vi "AlliGator Check whether Phasor Plot needs update.vi"(9 "Error In":errorcluster) -> (1 "Error Out":errorcluster)   [LabVIEW 2021, in "AlliGator Phasor Plot.lvlib"]
doc: "Checks whether any setting that could influence the Phasor Plot has been modified."
uses:
  AlliGator Phasor Plot.lvlib
  Settings/AlliGator Settings List.ctl
  AlliGator Phasor Plot Parameters v2.ctl
  Decay Analysis/Decay Preprocessing/AlliGator Decay Preprocessing Options.ctl
  Decay Analysis/Decay Preprocessing/AlliGator Background Subtraction Parameters.ctl
  Decay Analysis/Decay Preprocessing/AlliGator Baseline Subtraction Method.ctl
  Decay Analysis/Decay Preprocessing/AlliGator Decay Preprocessing Parameters.ctl
  Graphs/XY Graph/XY Graph Plot Shift Parameters.ctl
  Graphs/XY Graph/XY Graph Plot Shift Method.ctl
  Settings/AlliGator Low Count Pixels Rejection Options.ctl
  Settings/AlliGator High Count Pixels Rejection Options.ctl
  Settings/AlliGator Gate Arithmetic.ctl
  AlliGator Phasor Plot Smoothing Options.ctl
  Arrays/Kernel Type.ctl
  Arrays/Smoothing Algorithm.ctl
  AlliGator Phasor Plot Size.ctl
  Image/Named ROI Description.ctl
  Globals, Variables, Constants/AlliGator Variables List.ctl
  Phasor Calibration/AlliGator Phasor Calibration Options.ctl
  Phasor/Phasor Calibration Type.ctl
  Phasor Calibration/AlliGator Calibration Map Algorithm.ctl
  Variant/Variant to Data/Variant to Boolean.vi
  Variant/Variant to Data/Variant to I32.vi
  Settings/AlliGator Settings.lvlib
  GUI/AlliGator GUI.lvlib
  Decay Analysis/Decay Preprocessing/AlliGator Decay Preprocessing.lvlib
  Globals, Variables, Constants/AlliGator Globals, Variables & Constants.lvlib
  Graphs/XY Graph/XY Graph Add-Ons.lvlib
  Arrays/Arrays.lvlib
  Variant/Variant to Data/Variant to Data.lvlib
  Image/Image.lvlib
  Phasor Calibration/AlliGator Phasor Calibration.lvlib
  Phasor/Phasor.lvlib
panel:
  # "see the AlliGator License on the block diagram (Ctrl+E or Window:Show Block Diagram)"
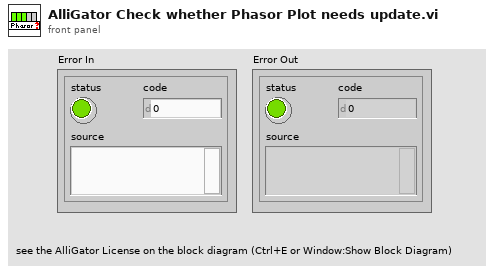
[diagram p1: front panel]
types:
  T1 = typedef "AlliGator Phasor Calibration.lvlib/AlliGator Phasor Calibration Options.ctl" = cluster{"Phasor Frequency":dbl[unit], "Phasor Calibration":cluster{"Calibration Lifetime":dbl[unit], "Calibration Type":T2, "Calibration Map Algorithm":T3, "Use Backup Calibration if needed":bool, "Backup Calibration Type":enum16{"Single Calibration", "Nearest Valid Calibration"}}}
  T2 = typedef "Phasor.lvlib/Phasor Calibration Type.ctl" = enum16{"None", "Single Phasor", "Phasor Series", "Phasor Map"}
  T3 = typedef "AlliGator Phasor Calibration.lvlib/AlliGator Calibration Map Algorithm.ctl" = enum16{"Simple Search", "Min Distance"}
  T4 = typedef "AlliGator Globals, Variables & Constants.lvlib/AlliGator Variables List.ctl" = enum16{"---- GUI ----", "GUI:Initialization Status", "GUI:State Indicators Refnum", "GUI:Original AlliGator Menu Items", "GUI:Current Action Loop State", "GUI:Script in progress", "GUI:Playback", "GUI:Loop Playback", "GUI:Search ROI Used", "GUI:Search ROI", "Decay Graph Max Legend Size", "Intensity Graph Max Legend Size", "Decay Statistics Graph Max Legend Size", "Phasor Graph Max Legend Size", "Phasor Ratio Graph Max Legend Size", "Lifetime Graph Max Legend Size", "---- Files ----", "Files:Export Dataset Frames as Individual Files", "Files:Show Batch Export Help Balloons", "Files:Frames in Dataset", "Files:ptu File Frame Start Indices", "Files:Current Frame in Dataset", "Files:Current Frame Timestamp", "Files:Dataset Loaded", "Files:Dataset Metadata", "Files:Dataset Channel", "Files:Dataset Data Description", "Files:Background Dataset Metadata", "Files:Background Dataset Channel", "Files:Background Dataset Data Description", "Files:Background File Subtraction", "Files:Background File Path", "Files:Background File Pile-up Correction", "Files:Background File Pixel Well Capacity", "Files:Background File Scaling Factor", "Files:Current Dataset Load Settings", "Files:Dataset Path", "Files:ICCD-specific Information", "Files:Macrotime Gate Separation", "------ Python Plugins ------", "Python Plugins:Information", "Python Plugins:Python Session", "Python Plugins:Valid Python Session?", "---- Source Image ----", "Source Image:ROIs", "Source Image:Current ROI", "Source Image:ROI Event Refnum", "X_Source Image Display Range", "X_Source Image Palette Information", "X_Type of Displayed Image", "X_Time Gate Slider", "Source Image:Palette List", "Source Image:Scale", "Source Image:ROI Overlay Color", "Source Image:Overlay to Erase", "Source Image:Is Displayed Image Accumulated", "Source Image:White Light Image Modified", "Source Image:Mask Image Modified", "---- Image Profile Window ----", "Image Profile:Window Event Refnum", "Image Profile:IntensityType", "Image Profile:Intensity Average Type", "Image Profile:Intensity-weighted SDV", "Image Profile:Box Profile Type", "Image Profile:Window Open", "Image Profile:Plotted Fit Parameter", "------ Phasor Graph -------", "Phasor Graph:Show Line", "---- Phasor Plot ---", "Phasor Plot:Parameters Changed", "Phasor Plot:FLI Dataset Modified since last Calculation", "Phasor Harmonics Data", "Selected Phasor Harmonics", "Phasor Harmonic Manager Event Refnum", "Phasor Plot:ROIs", "Phasor Plot:Current ROI", "Phasor Plot:ROI Event Refnum", "Phasor Plot:Image Reference Points", "Phasor Plot:Computed", "Phasor Plot:Palette Information", "Phasor Plot:Palette List", "Phasor Plot:Phasor Ratio Palette Information", "Phasor Plot:Phasor Ratio Palette List", "Phasor Plot:Image Scale", "Phasor Plot:Image Overlay to Erase", "Phasor Plot:Image Elements to Update", "Phasor Plot:Current Calculation Parameters", "Phasor Plot:Current Calibration Options", "Phasor Plot:Reset Cumulated Phasor Plot", "Phasor Plot:Reference 1", "Phasor Plot:Lifetime Reference 1", "Phasor Plot:Reference 1 Frequency", "Phasor Plot:Reference 2", "Phasor Plot:Lifetime Reference 2", "Phasor Plot:Reference 2 Frequency", "---- Decay Analysis ----", "Number of Selected Decays to Fit", "LS Fit Results", "LAR Fit Results", "BS Fit Results", "Last Decay Max - Min", "Best Fit Parameters", "Best Fit Parameter Names", "Actual Size X", "Actual Size Y", "Binning X", "Binning Y", "Actual # Gates", "Dataset Number", "Gates to...", "Gates Skipped", "Gates to keep", "Gate Step", "Gate Separation", "Reversed Gates", "Pile-up Correction", "Pixel Well Capacity", "Background Subtracted", "Background Subtraction Method", "Background Definition Range", "Background File (deprecated)", "Number of Dataset Accumulated", "Array of Accumulated Dataset Paths", "Do Averaged Datasets", "Destination File Path", "Process Plot Target", "Use 1/D as Phasor Frequency", "---- Decay Fit Parameter Map -----", "Decay Fit Parameter Map:Palette Information", "Decay Fit Parameter Map:Palette List", "---- Parameter Map ----", "Parameter Map:Palette Information", "Parameter Map:Palette List", "------- Local Decay Window ---------", "Local Decay Graph Window:Event Refnum", "Local Decay Graph Window:Use normalized IRF for convolution", "----- Miscellaneous ----", "Misc:Skippable Dialog Windows Status"}
  T5 = typedef "AlliGator Phasor Plot.lvlib/AlliGator Phasor Plot Parameters v2.ctl" = cluster{"Phasor Frequency":dbl[unit], "Decay Preprocessing Options & Parameters":T6, "FLI Dataset Modified":bool, "Source Image Settings":cluster{"Low Count Pixels Rejection Options":T12, "High Count Pixels Rejection Options":T13}, "Data Information":cluster{"Gate Width":dbl[unit], "Gate Separation":dbl[unit], "Step (Gate Separation)":i32, "Laser Period":dbl[unit], "SYNC Period":dbl[unit], "Channel Name":u16, "Channel Arithmetic":T14, "Pile-up Correction":bool, "Pixel Well Capacity":u32, "Dataset Scaling Factor":dbl}, "Phasor Plot":cluster{"Phasor Plot Smoothing Options":T15, "Phasor Plot Size":T18, "Selected Image ROI(s)":bool, "All Image ROIs":bool, "Selected Source Image ROI":i32, "Source Image ROIs":T19[]}}
  T6 = typedef "AlliGator Decay Preprocessing.lvlib/AlliGator Decay Preprocessing Options.ctl" = cluster{"Background Subtraction Parameters":T7, "Decay Preprocessing Parameters":T9, "Preprocessing Steps Order":string[]}
  T7 = typedef "AlliGator Decay Preprocessing.lvlib/AlliGator Background Subtraction Parameters.ctl" = cluster{"Background Definition Range":cluster{"Min Gate":dbl[unit], "Max Gate":dbl[unit]}, "Baseline Subtraction Method":T8, "Background Subtraction?":bool, "Background File":path, "Background Constant":dbl, "Background Scaling Factor":dbl, "Background Pile-up Correction":bool, "Background Pixel Well Capacity":u32}
  T8 = typedef "AlliGator Decay Preprocessing.lvlib/AlliGator Baseline Subtraction Method.ctl" = enum16{"Mean", "Min", "Square Gated Single-Exponential", "File", "Constant"}
  T9 = typedef "AlliGator Decay Preprocessing.lvlib/AlliGator Decay Preprocessing Parameters.ctl" = cluster{"Background Subtraction":bool, "Straighten Decay":bool, "Reverse Gates":bool, "1-Normalized Decay":bool, "Smoothen Decay":bool, "Smoothing Parameter":dbl, "Shift Decay":bool, "Decay Shift Parameters":T10, "Extrapolate Decay":bool, "Additional Points":u32, "Head Fraction":dbl, "Pixel-Normalize Decay":bool, "Use Periodicity":bool, "Use Cursors":bool, "Tail Fraction":dbl, "Use Decay Pre-Processing":bool, "Fold Decay":bool, "# Folds":u32, "[0-1]-Normalized Decay":bool}
  T10 = typedef "XY Graph Add-Ons.lvlib/XY Graph Plot Shift Parameters.ctl" = cluster{"Type":T11, "Shift":dbl[unit], "Threshold":dbl, "Rotate":bool}
  T11 = typedef "XY Graph Add-Ons.lvlib/XY Graph Plot Shift Method.ctl" = enum16{"Default", "CFD", "Threshold", "Cross-Correlation"}
  T12 = typedef "AlliGator Settings.lvlib/AlliGator Low Count Pixels Rejection Options.ctl" = cluster{"Background Low Threshold Factor":dbl, "Fixed Low Background Threshold":dbl, "Reject Low Count Pixels":bool, "Low Percentile":dbl}
  T13 = typedef "AlliGator Settings.lvlib/AlliGator High Count Pixels Rejection Options.ctl" = cluster{"Background High Threshold Factor":dbl, "Fixed High Background Threshold":dbl, "Reject High Count Pixels":bool, "High Percentile":dbl}
  T14 = typedef "AlliGator Settings.lvlib/AlliGator Gate Arithmetic.ctl" = enum16{"None", "INT-G2", "G2/INT*<INT>", "(1 - G2/INT)*<INT>"}
  T15 = typedef "AlliGator Phasor Plot.lvlib/AlliGator Phasor Plot Smoothing Options.ctl" = cluster{"Use Phasor Plot Smoothing":bool, "Kernel Type":T16, "Bin":i32, "Algorithm":T17}
  T16 = typedef "Arrays.lvlib/Kernel Type.ctl" = enum16{"Uniform", "Bilinear", "Gaussian"}
  T17 = typedef "Arrays.lvlib/Smoothing Algorithm.ctl" = enum16{"Rapid", "Thorough"}
  T18 = typedef "AlliGator Phasor Plot.lvlib/AlliGator Phasor Plot Size.ctl" = cluster{"H":i32, "V":i32, "Margin":dbl}
  T19 = typedef "Image.lvlib/Named ROI Description.ctl" = cluster{"ROI Descriptor":T20, "ROI Name":string, "Overlay Color":u32}
  T20 = typedef "ROI Descriptor" = cluster{"Global Rectangle":i32[], "Contours":cluster{"ID":enum32{"External", "Internal"}, "Type":u32, "Coordinates":i32[]}[]}
  T21 = typedef "AlliGator Settings.lvlib/AlliGator Settings List.ctl" = enum16{"GUI:Visible Settings Tab", "GUI:Last Run Version", "Source Image:Use Image Histogram for Contrast", "Source Image:Low Count Pixels Rejection Options", "Source Image:High Count Pixels Rejection Options", "Source Image:Use Image Brightness", "Source Image:Blend Overlay with Image Background", "Source Image:Use Fixed ROI Diameter", "Source Image:ROI Diameter", "Source Image:ROI Center Color", "Source Image:Peak Threshold", "Source Image:Intensity Threshold", "Source Image:Image Binning Options", "Source Image:Image Smoothing Options", "Source Image:Image Histogram Active", "Source Image:Invert Binary Mask", "Source Image:Hot Pixel Removal", "Source Image:Overlay Analyzed ROI Center", "Source Image:Auto-Adjust Contrast", "Source Image:Histogram Lower Percentile", "Source Image:Histogram Upper Percentile", "Source Image:Save Source Image", "Source Image:Scale Bar Options", "Source Image:Image Resolution (Pixel Size)", "Source Image:Flatfield Correction", "Source Image:Show Dead Left Columns Correction", "Source Image:Dead Left Columns Correction", "Source Image:Image Pre-Processing Operations Order", "Source Image:Overlay ROI Median", "Source Image:Median Overlay Color", "Data Information:Gate Width", "Data Information:Nanotime Gate Separation", "Data Information:Macrotime Gate Separation", "Data Information:Gate Step", "Data Information:# Gates", "Data Information:Gate Image Exposure", "Data Information:Gate Image Integration", "Data Information:Gates to Skip", "Data Information:Gates to Keep", "Data Information:Define Gates to", "Data Information:Channel Name", "Data Information:Available Channel Names", "Data Information:Channel Arithmetic", "Data Information:Background File Subtraction", "Data Information:Background File", "Data Information:Background Scaling Factor", "Data Information:Background Pile-up Correction", "Data Information:Background Pixel Well Capacity", "Data Information:Laser Period", "Data Information:SYNC Period", "Data Information:Pile-up Correction", "Data Information:Pixel Well Capacity", "Data Information:Dataset Scaling Factor", "Fluorescence Decay_Decay Pre-Processing:Reverse Gates", "Fluorescence Decay_Decay Pre-Processing:Verbose Decay Pre-Processing", "Fluorescence Decay_Decay Pre-Processing:Use Decay Pre-Processing", "Fluorescence Decay_Decay Pre-Processing:Background Subtraction", "Fluorescence Decay_Decay Pre-Processing:Background Definition Range", "Fluorescence Decay_Decay Pre-Processing:Baseline Subtraction Method", "Fluorescence Decay_Decay Pre-Processing:Decay Pre-Processing Operations Order", "Fluorescence Decay_Decay Pre-Processing:Smoothing Parameter", "Fluorescence Decay_Decay Pre-Processing:Shift Decay", "Fluorescence Decay_Decay Pre-Processing:Decay Shift Parameters", "Fluorescence Decay_Decay Pre-Processing:Fold Decay", "Fluorescence Decay_Decay Pre-Processing:# Folds", "Fluorescence Decay_Decay Pre-Processing:1-Normalize Decay", "Fluorescence Decay_Decay Pre-Processing:[0-1]-Normalize Decay", "Fluorescence Decay_Decay Pre-Processing:Smoothen Decay", "Fluorescence Decay_Decay Pre-Processing:Extrapolate Decay", "Fluorescence Decay_Decay Pre-Processing:Use Periodicity", "Fluorescence Decay_Decay Pre-Processing:Use Cursors", "Fluorescence Decay_Decay Pre-Processing:Tail Fraction", "Fluorescence Decay_Decay Pre-Processing:Head Fraction", "Fluorescence Decay_Decay Pre-Processing:Additional Points", "Fluorescence Decay_Decay Pre-Processing:Straighten Decay", "Fluorescence Decay_Decay Pre-Processing:Constant Background", "Fluorescence Decay_Decay Pre-Processing:Pixel-Normalize Decay", "Fluorescence Decay_Advanced Analysis:Extract IRF instead of Decay", "Fluorescence Decay_Advanced Analysis:IRF Extraction Options", "Fluorescence Decay_Advanced Analysis:IRF Optimization Options", "Fluorescence Decay_Advanced Analysis:Square Pulse Options", "Fluorescence Decay_Advanced Analysis:IRF Order", "Fluorescence Decay_Advanced Analysis:IRF Time Constants", "Fluorescence Decay_Advanced Analysis:Wavelet Analysis Options", "Fluorescence Decay_Advanced Analysis:Average Lifetime Options", "Fluorescence Decay_Fit Options:Fit Options", "Fluorescence Decay_Fit Options:Use Legacy Fitting Approach", "Fluorescence Decay_Fit Options:Use Data Information Laser Period", "Fluorescence Decay_Fit Parameters:Displayed Fit Parameters", "Fluorescence Decay_Fit Parameters:Fit Parameter Constraints", "Fluorescence Decay_Fit Parameters:Export Tabulated Results", "Fluorescence Decay_Fit Parameters:MLE Baseline Offset Type", "Fluorescence Decay_Fit Parameters:MLE Baseline Offset", "Fluorescence Decay_Fit Parameters:Guess Parameter Names", "Fluorescence Decay_Fit Parameters:Guess Parameter Values", "Fluorescence Decay_Fit Parameters:Guess Parameters Options", "Fluorescence Decay_Styles:Show Last Decay Only", "Fluorescence Decay_Styles:Decay Graph Color Array", "Fluorescence Decay:Decay Graph Active", "Fluorescence Decay Statistics:Min Peak Value", "Fluorescence Decay Statistics:Reject Low Decay Peak Pixels", "Fluorescence Decay Statistics:Reject High Decay Peak Pixels", "Fluorescence Decay Statistics:Max Peak Value", "Time Traces:Use File Timestamp", "Time Traces:Time Step", "Time Traces:Use Intensity Correction File", "Time Traces:Intensity Correction File", "Phasor Plot:Phasor Plot Smoothing Options", "Phasor Plot:Phasor Plot Size", "Phasor Plot:Phasor Plot Graphics Options", "Phasor Plot:Cumulative Phasor Plot", "Phasor Plot:Use Phasor Brightness", "Phasor Plot:Blend Overlay with Phasor Background", "Phasor Plot:Save Phasor Plot", "Phasor Plot:Show References", "Phasor Plot:Phasor Ratio Decay Range", "Phasor Plot:Exponential Fading", "Phasor Plot:Phasor Ratio Reference Colors", "Phasor Plot:Reference Radius", "Phasor Plot:Show Color Map Vertices", "Phasor Plot:Phasor Plot Active", "Phasor Plot:Phasor Ratio Color Map Type", "Phasor Plot:Phasor Ratio Color Map", "Phasor Plot:Phasor Ratio Display Range", "Phasor Plot:Selected Image ROI(s)", "Phasor Plot:All Image ROIs", "Phasor Plot:Selected Phasor Plot ROI(s)", "Phasor Plot:All Phasor Plot ROIs", "Phasor Plot:Phasor Ratio Color-Coded Quantity", "Phasor Plot:Store Phasor Harmonics", "Phasor Plot:Draw Reference Segment", "Phasor Plot:User-Defined Quantity", "Phasor Graph:Phasor Frequency", "Phasor Graph:Phasor Ratio Type", "Phasor Graph:Pixel-level Phasor Computation", "Phasor Graph:Save Phasor Graph", "Phasor Graph:Phasor Graph Active", "Phasor Graph:Phasor SDV Options", "Phasor Calibration:Use Backup Calibration if needed", "Phasor Graph:Define Shortest Lifetime as", "Phasor Calibration:Backup Calibration Type", "Phasor Calibration:Calibration Type", "Phasor Calibration:Calibration Lifetime", "Phasor Calibration:Calibration Map Algorithm", "Single-Exponential Phasor Locus (SEPL):Gate Parameters", "Single-Exponential Phasor Locus (SEPL):User-defined Gate", "Single-Exponential Phasor Locus (SEPL):User-defined IRF", "Single-Exponential Phasor Locus (SEPL):Phasor Parameters", "Single-Exponential Phasor Locus (SEPL):Decay & IRF Parameters", "Single-Exponential Phasor Locus (SEPL):Display Parameters", "Lifetime Analysis:Decay Analysis Parameters", "Lifetime Analysis:Lifetime Map Active", "Plugins:Python Settings", "Miscellaneous:Verbose Mode", "Miscellaneous:Beep after Script", "Miscellaneous:Saved Image File Format", "Miscellaneous:Exported Gate Image Settings", "Miscellaneous:Include Loading in Timing", "Miscellaneous:Verbose Settings Mode", "Miscellaneous:Histogram Options", "Miscellaneous:Beep on Error", "Miscellaneous:# Logical Processors Used", "Miscellaneous:ROI Description Max Characters", "Miscellaneous:Verbose Error Mode", "Miscellaneous:Transparent Mask Color"}
  T22 = enum16{"Single Calibration", "Nearest Valid Calibration"}
  T23 = cluster{"Min Gate":dbl[unit], "Max Gate":dbl[unit]}
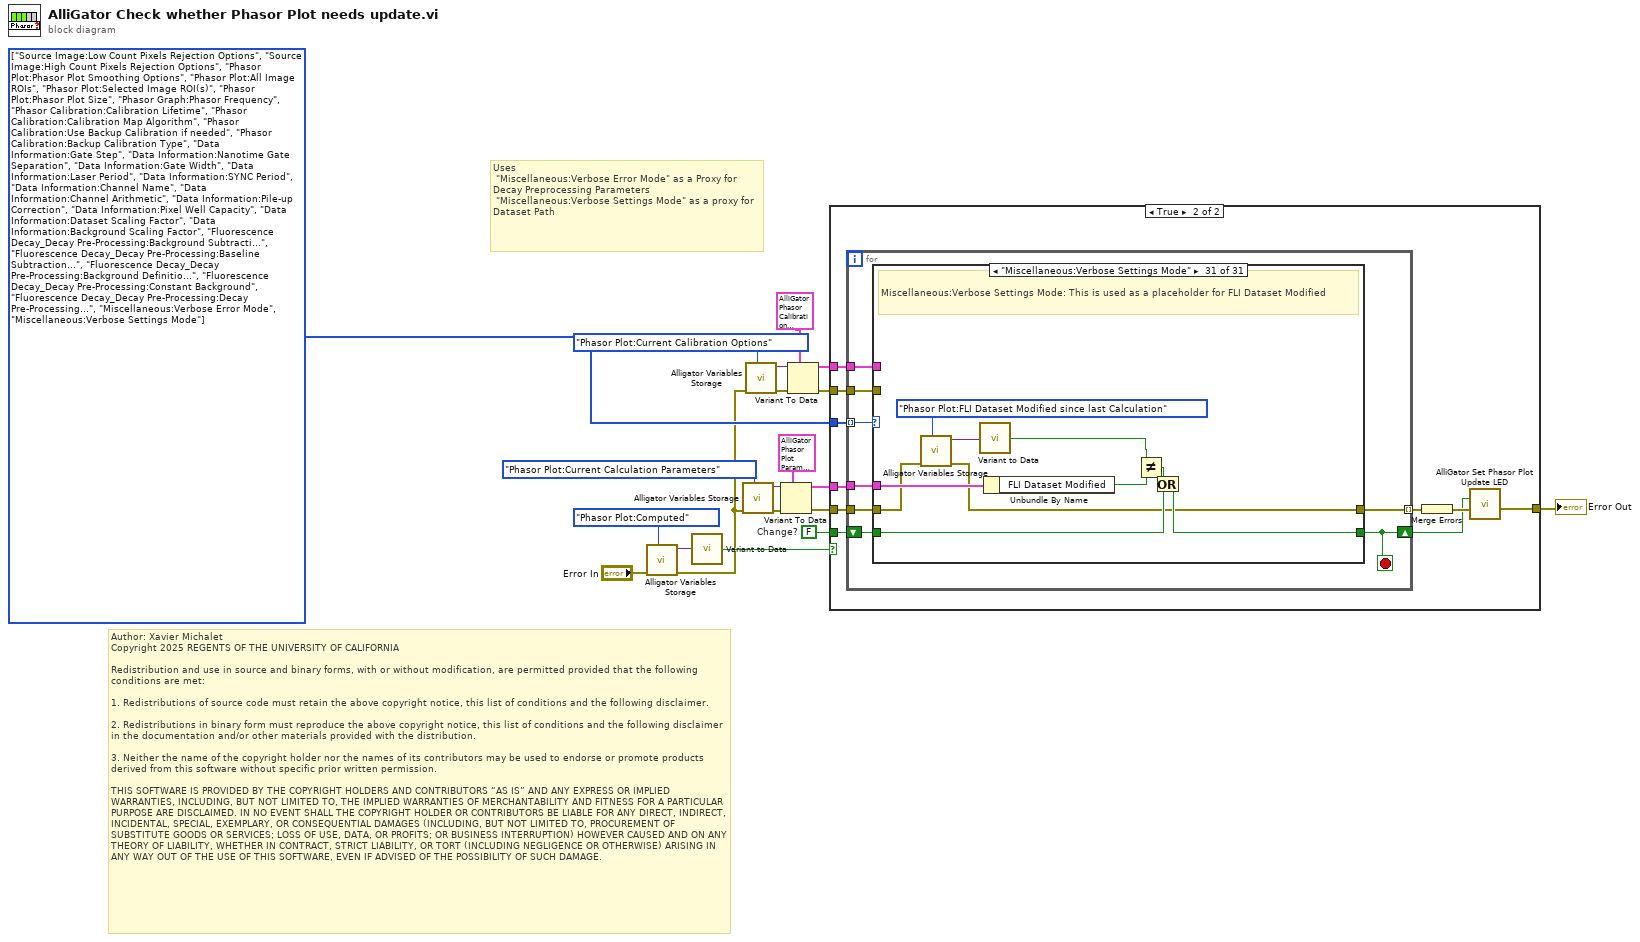
[diagram p0: block diagram]
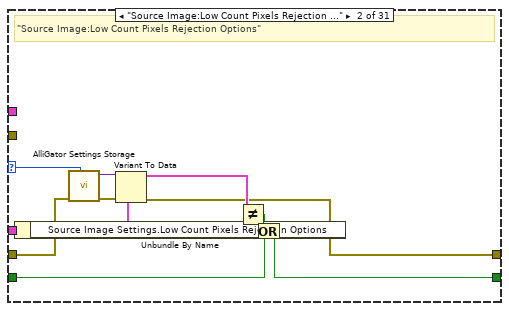
[diagram p4: hidden frame]
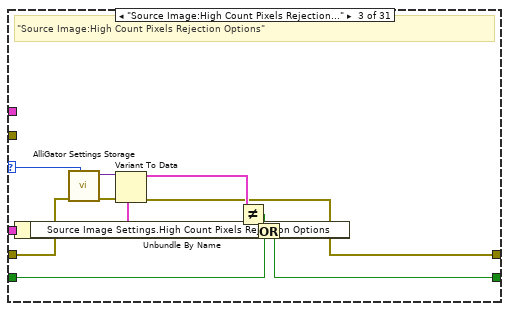
[diagram p5: hidden frame]
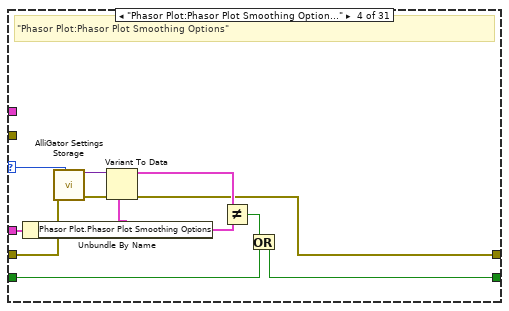
[diagram p6: hidden frame]
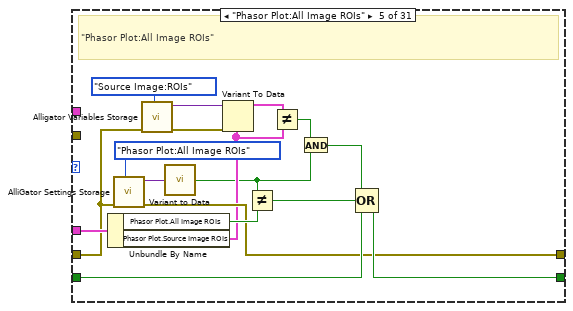
[diagram p7: hidden frame]
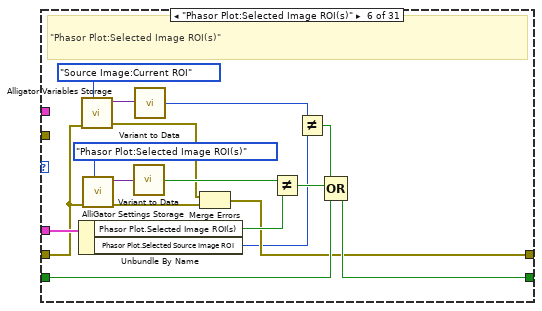
[diagram p8: hidden frame]
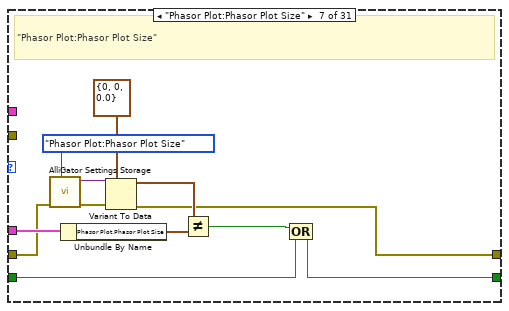
[diagram p9: hidden frame]
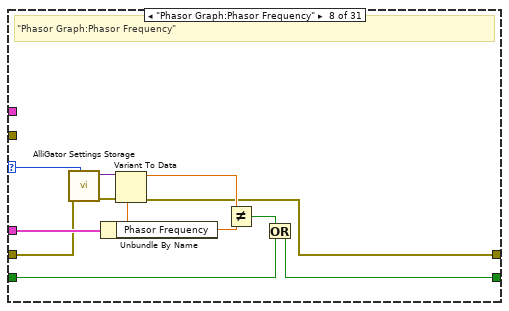
[diagram p10: hidden frame]
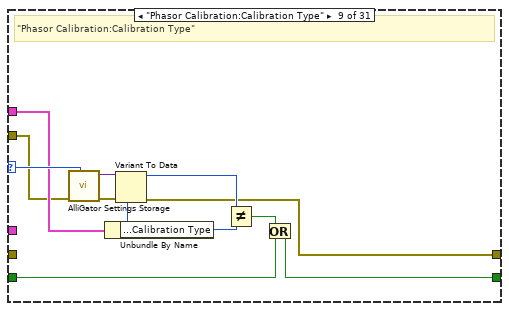
[diagram p11: hidden frame]
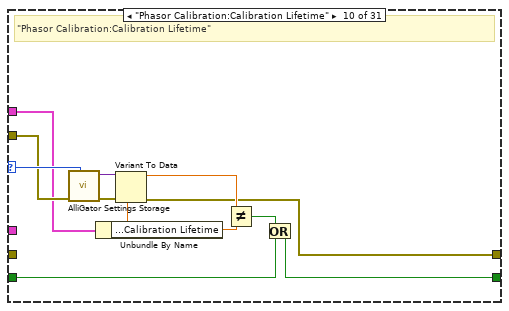
[diagram p12: hidden frame]
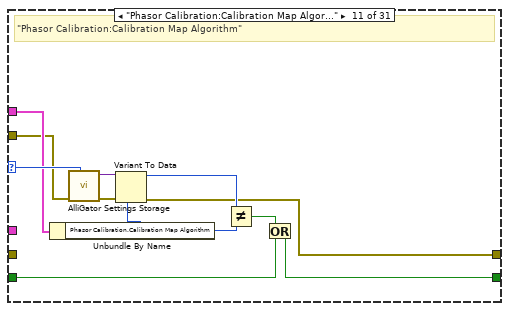
[diagram p13: hidden frame]
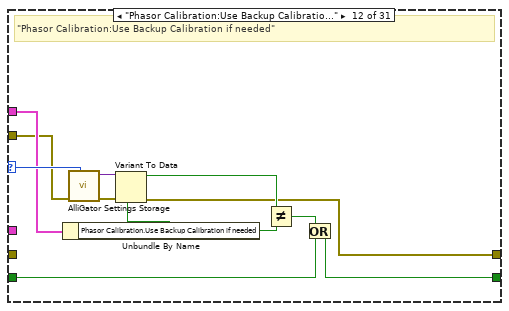
[diagram p14: hidden frame]
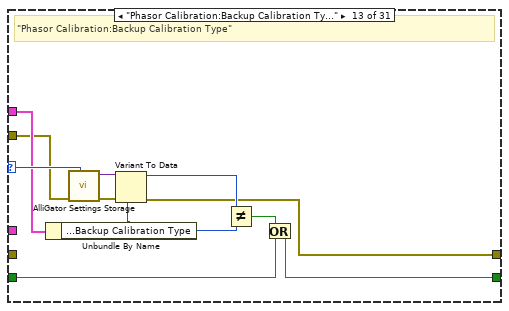
[diagram p15: hidden frame]
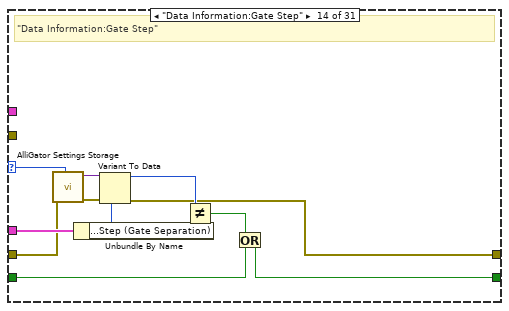
[diagram p16: hidden frame]
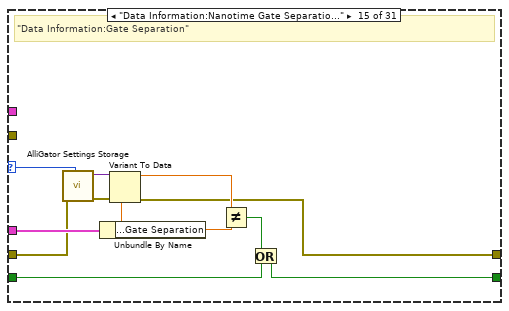
[diagram p17: hidden frame]
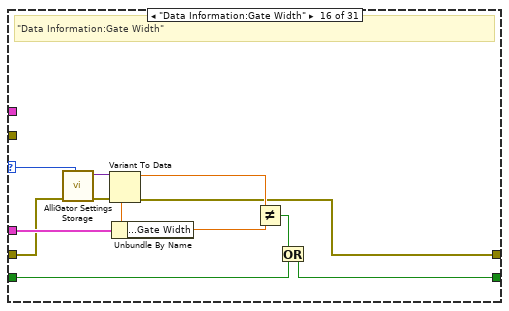
[diagram p18: hidden frame]
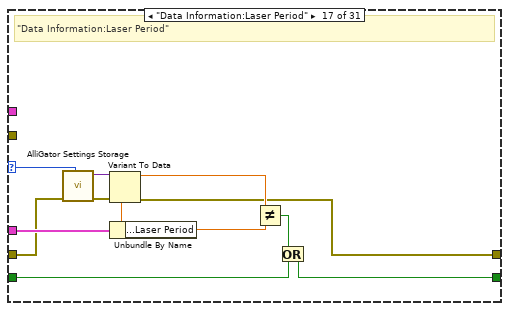
[diagram p19: hidden frame]
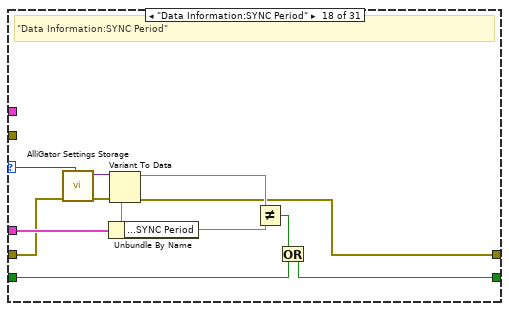
[diagram p20: hidden frame]
diagram:
  w13 = FALSE  # Change?
  w20 = T21[] [enum."Source Image:Low Count Pixels Rejection Options", enum."Source Image:High Count Pixels Rejection Options", enum."Phasor Plot:Phasor Plot Smoothing Options", enum."Phasor Plot:All Image ROIs", enum."Phasor Plot:Selected Image ROI(s)", enum."Phasor Plot:Phasor Plot Size", enum."Phasor Graph:Phasor Frequency", enum."Phasor Calibration:Calibration Lifetime", enum."Phasor Calibration:Calibration Map Algorithm", enum."Phasor Calibration:Use Backup Calibration if needed", enum."Phasor Calibration:Backup Calibration Type", enum."Data Information:Gate Step", enum."Data Information:Nanotime Gate Separation", enum."Data Information:Gate Width", enum."Data Information:Laser Period", enum."Data Information:SYNC Period", enum."Data Information:Channel Name", enum."Data Information:Channel Arithmetic", enum."Data Information:Pile-up Correction", enum."Data Information:Pixel Well Capacity", enum."Data Information:Dataset Scaling Factor", enum."Data Information:Background Scaling Factor", enum."Fluorescence Decay_Decay Pre-Processing:Background Subtraction", enum."Fluorescence Decay_Decay Pre-Processing:Baseline Subtraction Method", enum."Fluorescence Decay_Decay Pre-Processing:Background Definition Range", enum."Fluorescence Decay_Decay Pre-Processing:Constant Background", enum."Fluorescence Decay_Decay Pre-Processing:Decay Pre-Processing Operations Order", enum."Miscellaneous:Verbose Error Mode", enum."Miscellaneous:Verbose Settings Mode"] items=["GUI:Visible Settings Tab", "GUI:Last Run Version", "Source Image:Use Image Histogram for Contrast", "Source Image:Low Count Pixels Rejection Options", "Source Image:High Count Pixels Rejection Options", "Source Image:Use Image Brightness", "Source Image:Blend Overlay with Image Background", "Source Image:Use Fixed ROI Diameter", "Source Image:ROI Diameter", "Source Image:ROI Center Color", "Source Image:Peak Threshold", "Source Image:Intensity Threshold", "Source Image:Image Binning Options", "Source Image:Image Smoothing Options", "Source Image:Image Histogram Active", "Source Image:Invert Binary Mask", "Source Image:Hot Pixel Removal", "Source Image:Overlay Analyzed ROI Center", "Source Image:Auto-Adjust Contrast", "Source Image:Histogram Lower Percentile", "Source Image:Histogram Upper Percentile", "Source Image:Save Source Image", "Source Image:Scale Bar Options", "Source Image:Image Resolution (Pixel Size)", "Source Image:Flatfield Correction", "Source Image:Show Dead Left Columns Correction", "Source Image:Dead Left Columns Correction", "Source Image:Image Pre-Processing Operations Order", "Source Image:Overlay ROI Median", "Source Image:Median Overlay Color", "Data Information:Gate Width", "Data Information:Nanotime Gate Separation", "Data Information:Macrotime Gate Separation", "Data Information:Gate Step", "Data Information:# Gates", "Data Information:Gate Image Exposure", "Data Information:Gate Image Integration", "Data Information:Gates to Skip", "Data Information:Gates to Keep", "Data Information:Define Gates to", "Data Information:Channel Name", "Data Information:Available Channel Names", "Data Information:Channel Arithmetic", "Data Information:Background File Subtraction", "Data Information:Background File", "Data Information:Background Scaling Factor", "Data Information:Background Pile-up Correction", "Data Information:Background Pixel Well Capacity", "Data Information:Laser Period", "Data Information:SYNC Period", "Data Information:Pile-up Correction", "Data Information:Pixel Well Capacity", "Data Information:Dataset Scaling Factor", "Fluorescence Decay_Decay Pre-Processing:Reverse Gates", "Fluorescence Decay_Decay Pre-Processing:Verbose Decay Pre-Processing", "Fluorescence Decay_Decay Pre-Processing:Use Decay Pre-Processing", "Fluorescence Decay_Decay Pre-Processing:Background Subtraction", "Fluorescence Decay_Decay Pre-Processing:Background Definition Range", "Fluorescence Decay_Decay Pre-Processing:Baseline Subtraction Method", "Fluorescence Decay_Decay Pre-Processing:Decay Pre-Processing Operations Order", "Fluorescence Decay_Decay Pre-Processing:Smoothing Parameter", "Fluorescence Decay_Decay Pre-Processing:Shift Decay", "Fluorescence Decay_Decay Pre-Processing:Decay Shift Parameters", "Fluorescence Decay_Decay Pre-Processing:Fold Decay", "Fluorescence Decay_Decay Pre-Processing:# Folds", "Fluorescence Decay_Decay Pre-Processing:1-Normalize Decay", "Fluorescence Decay_Decay Pre-Processing:[0-1]-Normalize Decay", "Fluorescence Decay_Decay Pre-Processing:Smoothen Decay", "Fluorescence Decay_Decay Pre-Processing:Extrapolate Decay", "Fluorescence Decay_Decay Pre-Processing:Use Periodicity", "Fluorescence Decay_Decay Pre-Processing:Use Cursors", "Fluorescence Decay_Decay Pre-Processing:Tail Fraction", "Fluorescence Decay_Decay Pre-Processing:Head Fraction", "Fluorescence Decay_Decay Pre-Processing:Additional Points", "Fluorescence Decay_Decay Pre-Processing:Straighten Decay", "Fluorescence Decay_Decay Pre-Processing:Constant Background", "Fluorescence Decay_Decay Pre-Processing:Pixel-Normalize Decay", "Fluorescence Decay_Advanced Analysis:Extract IRF instead of Decay", "Fluorescence Decay_Advanced Analysis:IRF Extraction Options", "Fluorescence Decay_Advanced Analysis:IRF Optimization Options", "Fluorescence Decay_Advanced Analysis:Square Pulse Options", "Fluorescence Decay_Advanced Analysis:IRF Order", "Fluorescence Decay_Advanced Analysis:IRF Time Constants", "Fluorescence Decay_Advanced Analysis:Wavelet Analysis Options", "Fluorescence Decay_Advanced Analysis:Average Lifetime Options", "Fluorescence Decay_Fit Options:Fit Options", "Fluorescence Decay_Fit Options:Use Legacy Fitting Approach", "Fluorescence Decay_Fit Options:Use Data Information Laser Period", "Fluorescence Decay_Fit Parameters:Displayed Fit Parameters", "Fluorescence Decay_Fit Parameters:Fit Parameter Constraints", "Fluorescence Decay_Fit Parameters:Export Tabulated Results", "Fluorescence Decay_Fit Parameters:MLE Baseline Offset Type", "Fluorescence Decay_Fit Parameters:MLE Baseline Offset", "Fluorescence Decay_Fit Parameters:Guess Parameter Names", "Fluorescence Decay_Fit Parameters:Guess Parameter Values", "Fluorescence Decay_Fit Parameters:Guess Parameters Options", "Fluorescence Decay_Styles:Show Last Decay Only", "Fluorescence Decay_Styles:Decay Graph Color Array", "Fluorescence Decay:Decay Graph Active", "Fluorescence Decay Statistics:Min Peak Value", "Fluorescence Decay Statistics:Reject Low Decay Peak Pixels", "Fluorescence Decay Statistics:Reject High Decay Peak Pixels", "Fluorescence Decay Statistics:Max Peak Value", "Time Traces:Use File Timestamp", "Time Traces:Time Step", "Time Traces:Use Intensity Correction File", "Time Traces:Intensity Correction File", "Phasor Plot:Phasor Plot Smoothing Options", "Phasor Plot:Phasor Plot Size", "Phasor Plot:Phasor Plot Graphics Options", "Phasor Plot:Cumulative Phasor Plot", "Phasor Plot:Use Phasor Brightness", "Phasor Plot:Blend Overlay with Phasor Background", "Phasor Plot:Save Phasor Plot", "Phasor Plot:Show References", "Phasor Plot:Phasor Ratio Decay Range", "Phasor Plot:Exponential Fading", "Phasor Plot:Phasor Ratio Reference Colors", "Phasor Plot:Reference Radius", "Phasor Plot:Show Color Map Vertices", "Phasor Plot:Phasor Plot Active", "Phasor Plot:Phasor Ratio Color Map Type", "Phasor Plot:Phasor Ratio Color Map", "Phasor Plot:Phasor Ratio Display Range", "Phasor Plot:Selected Image ROI(s)", "Phasor Plot:All Image ROIs", "Phasor Plot:Selected Phasor Plot ROI(s)", "Phasor Plot:All Phasor Plot ROIs", "Phasor Plot:Phasor Ratio Color-Coded Quantity", "Phasor Plot:Store Phasor Harmonics", "Phasor Plot:Draw Reference Segment", "Phasor Plot:User-Defined Quantity", "Phasor Graph:Phasor Frequency", "Phasor Graph:Phasor Ratio Type", "Phasor Graph:Pixel-level Phasor Computation", "Phasor Graph:Save Phasor Graph", "Phasor Graph:Phasor Graph Active", "Phasor Graph:Phasor SDV Options", "Phasor Calibration:Use Backup Calibration if needed", "Phasor Graph:Define Shortest Lifetime as", "Phasor Calibration:Backup Calibration Type", "Phasor Calibration:Calibration Type", "Phasor Calibration:Calibration Lifetime", "Phasor Calibration:Calibration Map Algorithm", "Single-Exponential Phasor Locus (SEPL):Gate Parameters", "Single-Exponential Phasor Locus (SEPL):User-defined Gate", "Single-Exponential Phasor Locus (SEPL):User-defined IRF", "Single-Exponential Phasor Locus (SEPL):Phasor Parameters", "Single-Exponential Phasor Locus (SEPL):Decay & IRF Parameters", "Single-Exponential Phasor Locus (SEPL):Display Parameters", "Lifetime Analysis:Decay Analysis Parameters", "Lifetime Analysis:Lifetime Map Active", "Plugins:Python Settings", "Miscellaneous:Verbose Mode", "Miscellaneous:Beep after Script", "Miscellaneous:Saved Image File Format", "Miscellaneous:Exported Gate Image Settings", "Miscellaneous:Include Loading in Timing", "Miscellaneous:Verbose Settings Mode", "Miscellaneous:Histogram Options", "Miscellaneous:Beep on Error", "Miscellaneous:# Logical Processors Used", "Miscellaneous:ROI Description Max Characters", "Miscellaneous:Verbose Error Mode", "Miscellaneous:Transparent Mask Color"] ("Array")
  # "Author: Xavier Michalet\nCopyright 2025 REGENTS OF THE UNIVERSITY OF CALIFORNIA\n\nRedistribution and use in source and binary forms, with or without modification, are permitted provided that the following conditions are met:\n\n1. Redistributions of source code must retain the above copyright notice, this list of conditions and the following disclaimer.\n\n2. Redistributions in binary form must reproduce the above copyright notice, this list of conditions and the following disclaimer in the documentation and/or other materials provided with the distribution.\n\n3. Neither the name of the copyright holder nor the names of its contributors may be used to endorse or promote products derived from this software without specific prior written permission.\n\nTHIS SOFTWARE IS PROVIDED BY THE COPYRIGHT HOLDERS AND CONTRIBUTORS “AS IS” AND ANY EXPRESS OR IMPLIED WARRANTIES, INCLUDING, BUT NOT LIMITED TO, THE IMPLIED WARRANTIES OF MERCHANTABILITY AND FITNESS FOR A PARTICULAR PURPOSE ARE DISCLAIMED. IN NO EVENT SHALL THE COPYRIGHT HOLDER OR CONTRIBUTORS BE LIABLE FOR ANY DIRECT, INDIRECT, INCIDENTAL, SPECIAL, EXEMPLARY, OR CONSEQUENTIAL DAMAGES (INCLUDING, BUT NOT LIMITED TO, PROCUREMENT OF SUBSTITUTE GOODS OR SERVICES; LOSS OF USE, DATA, OR PROFITS; OR BUSINESS INTERRUPTION) HOWEVER CAUSED AND ON ANY THEORY OF LIABILITY, WHETHER IN CONTRACT, STRICT LIABILITY, OR TORT (INCLUDING NEGLIGENCE OR OTHERWISE) ARISING IN ANY WAY OUT OF THE USE OF THIS SOFTWARE, EVEN IF ADVISED OF THE POSSIBILITY OF SUCH DAMAGE."
  # "Uses\n \"Miscellaneous:Verbose Error Mode\" as a Proxy for Decay Preprocessing Parameters\n \"Miscellaneous:Verbose Settings Mode\" as a proxy for Dataset Path"
  n1 = call "Alligator Variables Storage.vi"("AlliGator Variable"=AlliGator_Variables_List."Phasor Plot:Computed" ("Alligator Variable"), "Error In"="Error In") -> ("Error Out"=w6:errorcluster, "Data out"=w10:variant)  [unwired: 7 in, 1 out]
  n2 = call-poly "Variant to Data.vi"("Variant"=w10) -> ("Value"=w9:bool)  [unwired: 8 in]
  n3 = call "Alligator Variables Storage.vi"("AlliGator Variable"=AlliGator_Variables_List."Phasor Plot:Current Calculation Parameters" ("Alligator Variable"), "Error In"=w6) -> ("Error Out"=w17:errorcluster, "Data out"=w18:variant)  [unwired: 7 in, 1 out]
  n4 = call "Alligator Variables Storage.vi"("AlliGator Variable"=AlliGator_Variables_List."Phasor Plot:Current Calibration Options" ("Alligator Variable"), "Error In"=w6) -> ("Error Out"=w5:errorcluster, "Data out"=w4:variant)  [unwired: 7 in, 1 out]
  n5 = Variant To Data(error in=w17, type=T5 {"Phasor Frequency"=0.0, "Decay Preprocessing Options & Parameters"={"Background Subtraction Parameters"={"Background Definition Range"={"Min Gate"=0.0, "Max Gate"=0.0}, "Baseline Subtraction Method"=enum."Mean", "Background Subtraction?"=FALSE, "Background File"=path "", "Background Constant"=0.0, "Background Scaling Factor"=1.0, "Background Pile-up Correction"=FALSE, "Background Pixel Well Capacity"=1}, "Decay Preprocessing Parameters"={"Background Subtraction"=FALSE, "Straighten Decay"=FALSE, "Reverse Gates"=FALSE, "1-Normalized Decay"=FALSE, "Smoothen Decay"=FALSE, "Smoothing Parameter"=0.0, "Shift Decay"=FALSE, "Decay Shift Parameters"={"Type"=enum."Default", "Shift"=0.0, "Threshold"=0.0, "Rotate"=FALSE}, "Extrapolate Decay"=FALSE, "Additional Points"=0, "Head Fraction"=0.0, "Pixel-Normalize Decay"=FALSE, "Use Periodicity"=FALSE, "Use Cursors"=FALSE, "Tail Fraction"=0.0, "Use Decay Pre-Processing"=TRUE, "Fold Decay"=FALSE, "# Folds"=1, "[0-1]-Normalized Decay"=FALSE}, "Preprocessing Steps Order"=[]}, "FLI Dataset Modified"=FALSE, "Source Image Settings"={"Low Count Pixels Rejection Options"={"Background Low Threshold Factor"=0.0, "Fixed Low Background Threshold"=0.0, "Reject Low Count Pixels"=FALSE, "Low Percentile"=0.0}, "High Count Pixels Rejection Options"={"Background High Threshold Factor"=0.0, "Fixed High Background Threshold"=20000.0, "Reject High Count Pixels"=FALSE, "High Percentile"=100.0}}, "Data Information"={"Gate Width"=0.0, "Gate Separation"=0.0, "Step (Gate Separation)"=0, "Laser Period"=0.0, "SYNC Period"=0.0, "Channel Name"=0, "Channel Arithmetic"=enum."None", "Pile-up Correction"=FALSE, "Pixel Well Capacity"=1, "Dataset Scaling Factor"=1.0}, "Phasor Plot"={"Phasor Plot Smoothing Options"={"Use Phasor Plot Smoothing"=FALSE, "Kernel Type"=enum."Uniform", "Bin"=1, "Algorithm"=enum."Rapid"}, "Phasor Plot Size"={"H"=0, "V"=0, "Margin"=0.0}, "Selected Image ROI(s)"=FALSE, "All Image ROIs"=FALSE, "Selected Source Image ROI"=0, "Source Image ROIs"=[]}} ("TG Phasor Plot Parameters"), Variant=w18) -> (data=w12:T5, error out=w16:errorcluster)
  n6 = Variant To Data(error in=w5, type=T1 {"Phasor Frequency"=0.0, "Phasor Calibration"={"Calibration Lifetime"=1e-09, "Calibration Type"=enum."Single Phasor", "Calibration Map Algorithm"=enum."Simple Search", "Use Backup Calibration if needed"=TRUE, "Backup Calibration Type"=enum."Single Calibration"}} ("AlliGator Phasor Calibration Options"), Variant=w4) -> (data=w2:T1, error out=w1:errorcluster)
  n7 = case shown="True" w9 {
    tunnel: w20 -> [_ w31]
    tunnel: [w21 w30] -> w19
    tunnel: w16 -> [w21 w27]
    tunnel: w13 -> [_ w28]
    tunnel: w12 -> [_ w29]
    tunnel: w2 -> [_ w23]
    tunnel: w1 -> [_ w22]
    frame False {
      # "if not phasor plot computed, parameters can change without turning on the LED"
    }
    frame True {
      n8 = for {
        tunnel: w29 -> [w39]
        tunnel: w27 -> [w38]
        tunnel: w31 -> [w35] mode=indexing
        shift-right: [w34] -> w24
        shift-left: w28 -> [w37]
        tunnel: [w36] -> w26 mode=indexing
        tunnel: w23 -> [w33]
        tunnel: w22 -> [w32]
        stop <- w34 stop-if-true
        n9 = case shown="\"Miscellaneous:Verbose Settings Mode\"" w35 {
          selector: w35 -> [_ w43 w54 w70 _ _ _ w122 w136 w147 w158 w169 w180 w188 w207 w218 w229 w240 w251 w262 w273 w284 w295 w298 w309 w320 w331 w342 w353 _ _]
          tunnel: w39 -> [_ w47 w58 w71 w90 w107 w120 w126 _ _ _ _ _ w192 w208 w219 w230 w241 w252 w263 w274 w285 w296 w302 w313 w324 w335 w346 w357 w369 w380]
          tunnel: w38 -> [w41 w42 w53 w72 w82 w98 w116 w125 _ _ _ _ _ w191 w206 w217 w228 w239 w250 w261 w272 w283 w294 w297 w308 w319 w330 w341 w352 w365 w376]
          tunnel: w37 -> [w40 w45 w56 w73 w89 w106 w119 w123 w137 w148 w159 w170 w181 w189 w200 w211 w222 w233 w244 w255 w266 w277 w288 w300 w311 w322 w333 w344 w355 w368 w379]
          tunnel: [w40 w44 w55 w64 w88 w105 w118 w121 w135 w146 w157 w168 w179 w187 w198 w209 w220 w231 w242 w253 w264 w275 w286 w299 w310 w321 w332 w343 w354 w367 w378] -> w34
          tunnel: [w41 w46 w57 w65 w86 w96 w109 w124 w138 w149 w160 w171 w182 w190 w199 w210 w221 w232 w243 w254 w265 w276 w287 w301 w312 w323 w334 w345 w356 w364 w377] -> w36
          tunnel: w33 -> [_ _ _ _ _ _ _ _ w133 w143 w155 w166 w177 _ _ _ _ _ _ _ _ _ _ _ _ _ _ _ _ _ _]
          tunnel: w32 -> [_ _ _ _ _ _ _ _ w132 w144 w154 w165 w176 _ _ _ _ _ _ _ _ _ _ _ _ _ _ _ _ _ _]
          frame "GUI:Visible Settings Tab", Default {
            # "\"GUI:Visible Settings Tab\", Default"
          }
          frame "Source Image:Low Count Pixels Rejection Options" {
            # "\"Source Image:Low Count Pixels Rejection Options\""
            n10 = Unbundle By Name(w47) -> ("Source Image Settings.Low Count Pixels Rejection Options"=w50:T12)
            n11 = call "AlliGator Settings Storage.vi"("AlliGator Settings List"=w43, "Error In"=w42) -> ("Error Out"=w51:errorcluster, "Variant Data out"=w52:variant)  [unwired: 8 in]
            n12 = Variant To Data(error in=w51, type=w50, Variant=w52) -> (data=w49:T12, error out=w46:errorcluster)
            n13 = Not Equal?(x=w49, y=w50) -> (x != y?=w48:bool)
            n14 = Or(x=w48, y=w45) -> (x .or. y?=w44:bool)
          }
          frame "Source Image:High Count Pixels Rejection Options" {
            # "\"Source Image:High Count Pixels Rejection Options\""
            n15 = Unbundle By Name(w58) -> ("Source Image Settings.High Count Pixels Rejection Options"=w61:T13)
            n16 = call "AlliGator Settings Storage.vi"("AlliGator Settings List"=w54, "Error In"=w53) -> ("Error Out"=w62:errorcluster, "Variant Data out"=w63:variant)  [unwired: 8 in]
            n17 = Variant To Data(error in=w62, type=w61, Variant=w63) -> (data=w60:T13, error out=w57:errorcluster)
            n18 = Not Equal?(x=w60, y=w61) -> (x != y?=w59:bool)
            n19 = Or(x=w59, y=w56) -> (x .or. y?=w55:bool)
          }
          frame "Phasor Plot:Phasor Plot Smoothing Options" {
            # "\"Phasor Plot:Phasor Plot Smoothing Options\""
            n20 = Unbundle By Name(w71) -> ("Phasor Plot.Phasor Plot Smoothing Options"=w67:T15)
            n21 = call "AlliGator Settings Storage.vi"("AlliGator Settings List"=w70, "Error In"=w72) -> ("Error Out"=w69:errorcluster, "Variant Data out"=w66:variant)  [unwired: 8 in]
            n22 = Variant To Data(error in=w69, type=w67, Variant=w66) -> (data=w68:T15, error out=w65:errorcluster)
            n23 = Not Equal?(x=w68, y=w67) -> (x != y?=w74:bool)
            n24 = Or(x=w74, y=w73) -> (x .or. y?=w64:bool)
          }
          frame "Phasor Plot:All Image ROIs" {
            # "\"Phasor Plot:All Image ROIs\""
            n25 = Unbundle By Name(w90) -> ("Phasor Plot.All Image ROIs"=w87:bool, "Phasor Plot.Source Image ROIs"=w78:T19[])
            n26 = call "AlliGator Settings Storage.vi"("AlliGator Settings List"=AlliGator_Settings_List."Phasor Plot:All Image ROIs", "Error In"=w82) -> ("Error Out"=w86:errorcluster, "Variant Data out"=w85:variant)  [unwired: 8 in]
            n27 = call "Alligator Variables Storage.vi"("AlliGator Variable"=AlliGator_Variables_List."Source Image:ROIs" ("Alligator Variable"), "Error In"=w82) -> ("Error Out"=w80:errorcluster, "Data out"=w81:variant)  [unwired: 7 in, 1 out]
            n28 = call-poly "Variant to Data.vi"("Variant"=w85) -> ("Value"=w76:bool)  [unwired: 8 in]
            n29 = Variant To Data(error in=w80, type=w78, Variant=w81) -> (data=w79:T19[])  [unwired: 1 out]
            n30 = Not Equal?(x=w76, y=w87) -> (x != y?=w91:bool)
            n31 = Not Equal?(x=w79, y=w78) -> (x != y?=w77:bool)
            n32 = And(x=w77, y=w76) -> (x .and. y?=w75:bool)
            n33 = Compound Arithmetic op=OR(w75, w91, w89) -> (w88:bool)
          }
          frame "Phasor Plot:Selected Image ROI(s)" {
            # "\"Phasor Plot:Selected Image ROI(s)\""
            n34 = Unbundle By Name(w107) -> ("Phasor Plot.Selected Image ROI(s)"=w103:bool, "Phasor Plot.Selected Source Image ROI"=w93:i32)
            n35 = call "Alligator Variables Storage.vi"("AlliGator Variable"=AlliGator_Variables_List."Source Image:Current ROI" ("Alligator Variable"), "Error In"=w98) -> ("Error Out"=w95:errorcluster, "Data out"=w97:variant)  [unwired: 7 in, 1 out]
            n36 = call "AlliGator Settings Storage.vi"("AlliGator Settings List"=AlliGator_Settings_List."Phasor Plot:Selected Image ROI(s)", "Error In"=w98) -> ("Error Out"=w102:errorcluster, "Variant Data out"=w101:variant)  [unwired: 8 in]
            n37 = call-poly "Variant to Data.vi"("Variant"=w101) -> ("Value"=w104:bool)  [unwired: 8 in]
            n38 = call-poly "Variant to Data.vi"("Variant"=w97) -> ("Value"=w94:i32)  [unwired: 8 in]
            n39 = Merge Errors(w95, w102) -> (w96:errorcluster)
            n40 = Not Equal?(x=w104, y=w103) -> (x != y?=w108:bool)
            n41 = Not Equal?(x=w94, y=w93) -> (x != y?=w92:bool)
            n42 = Compound Arithmetic op=OR(w92, w108, w106) -> (w105:bool)
          }
          frame "Phasor Plot:Phasor Plot Size" {
            # "\"Phasor Plot:Phasor Plot Size\""
            n43 = call "AlliGator Settings Storage.vi"("AlliGator Settings List"=AlliGator_Settings_List."Phasor Plot:Phasor Plot Size", "Error In"=w116) -> ("Error Out"=w115:errorcluster, "Variant Data out"=w114:variant)  [unwired: 8 in]
            n44 = Unbundle By Name(w120) -> ("Phasor Plot.Phasor Plot Size"=w111:T18)
            n45 = Variant To Data(error in=w115, type=T18 {"H"=0, "V"=0, "Margin"=0.0} ("Phasor Plot Size"), Variant=w114) -> (data=w112:T18, error out=w109:errorcluster)
            n46 = Not Equal?(x=w112, y=w111) -> (x != y?=w110:bool)
            n47 = Compound Arithmetic op=OR(w110, w119) -> (w118:bool)
          }
          frame "Phasor Graph:Phasor Frequency" {
            # "\"Phasor Graph:Phasor Frequency\""
            n48 = call "AlliGator Settings Storage.vi"("AlliGator Settings List"=w122, "Error In"=w125) -> ("Error Out"=w130:errorcluster, "Variant Data out"=w131:variant)  [unwired: 8 in]
            n49 = Unbundle By Name(w126) -> ("Phasor Frequency"=w129:dbl[unit])
            n50 = Variant To Data(error in=w130, type=w129, Variant=w131) -> (data=w128:dbl[unit], error out=w124:errorcluster)
            n51 = Not Equal?(x=w128, y=w129) -> (x != y?=w127:bool)
            n52 = Or(x=w127, y=w123) -> (x .or. y?=w121:bool)
          }
          frame "Phasor Calibration:Calibration Type" {
            # "\"Phasor Calibration:Calibration Type\""
            n53 = call "AlliGator Settings Storage.vi"("AlliGator Settings List"=w136, "Error In"=w132) -> ("Error Out"=w141:errorcluster, "Variant Data out"=w142:variant)  [unwired: 8 in]
            n54 = Unbundle By Name(w133) -> ("Phasor Calibration.Calibration Type"=w134:T2)
            n55 = Variant To Data(error in=w141, type=w134, Variant=w142) -> (data=w140:T2, error out=w138:errorcluster)
            n56 = Not Equal?(x=w140, y=w134) -> (x != y?=w139:bool)
            n57 = Or(x=w139, y=w137) -> (x .or. y?=w135:bool)
          }
          frame "Phasor Calibration:Calibration Lifetime" {
            # "\"Phasor Calibration:Calibration Lifetime\""
            n58 = call "AlliGator Settings Storage.vi"("AlliGator Settings List"=w147, "Error In"=w144) -> ("Error Out"=w152:errorcluster, "Variant Data out"=w153:variant)  [unwired: 8 in]
            n59 = Unbundle By Name(w143) -> ("Phasor Calibration.Calibration Lifetime"=w145:dbl[unit])
            n60 = Variant To Data(error in=w152, type=w145, Variant=w153) -> (data=w151:dbl[unit], error out=w149:errorcluster)
            n61 = Not Equal?(x=w151, y=w145) -> (x != y?=w150:bool)
            n62 = Or(x=w150, y=w148) -> (x .or. y?=w146:bool)
          }
          frame "Phasor Calibration:Calibration Map Algorithm" {
            # "\"Phasor Calibration:Calibration Map Algorithm\""
            n63 = Unbundle By Name(w155) -> ("Phasor Calibration.Calibration Map Algorithm"=w156:T3)
            n64 = call "AlliGator Settings Storage.vi"("AlliGator Settings List"=w158, "Error In"=w154) -> ("Error Out"=w163:errorcluster, "Variant Data out"=w164:variant)  [unwired: 8 in]
            n65 = Variant To Data(error in=w163, type=w156, Variant=w164) -> (data=w162:T3, error out=w160:errorcluster)
            n66 = Not Equal?(x=w162, y=w156) -> (x != y?=w161:bool)
            n67 = Or(x=w161, y=w159) -> (x .or. y?=w157:bool)
          }
          frame "Phasor Calibration:Use Backup Calibration if needed" {
            # "\"Phasor Calibration:Use Backup Calibration if needed\""
            n68 = Unbundle By Name(w166) -> ("Phasor Calibration.Use Backup Calibration if needed"=w167:bool)
            n69 = call "AlliGator Settings Storage.vi"("AlliGator Settings List"=w169, "Error In"=w165) -> ("Error Out"=w174:errorcluster, "Variant Data out"=w175:variant)  [unwired: 8 in]
            n70 = Variant To Data(error in=w174, type=w167, Variant=w175) -> (data=w173:bool, error out=w171:errorcluster)
            n71 = Not Equal?(x=w173, y=w167) -> (x != y?=w172:bool)
            n72 = Or(x=w172, y=w170) -> (x .or. y?=w168:bool)
          }
          frame "Phasor Calibration:Backup Calibration Type" {
            # "\"Phasor Calibration:Backup Calibration Type\""
            n73 = Unbundle By Name(w177) -> ("Phasor Calibration.Backup Calibration Type"=w178:T22)
            n74 = call "AlliGator Settings Storage.vi"("AlliGator Settings List"=w180, "Error In"=w176) -> ("Error Out"=w185:errorcluster, "Variant Data out"=w186:variant)  [unwired: 8 in]
            n75 = Variant To Data(error in=w185, type=w178, Variant=w186) -> (data=w184:T22, error out=w182:errorcluster)
            n76 = Not Equal?(x=w184, y=w178) -> (x != y?=w183:bool)
            n77 = Or(x=w183, y=w181) -> (x .or. y?=w179:bool)
          }
          frame "Data Information:Gate Step" {
            # "\"Data Information:Gate Step\""
            n78 = call "AlliGator Settings Storage.vi"("AlliGator Settings List"=w188, "Error In"=w191) -> ("Error Out"=w194:errorcluster, "Variant Data out"=w193:variant)  [unwired: 8 in]
            n79 = Unbundle By Name(w192) -> ("Data Information.Step (Gate Separation)"=w195:i32)
            n80 = Variant To Data(error in=w194, type=w195, Variant=w193) -> (data=w196:i32, error out=w190:errorcluster)
            n81 = Not Equal?(x=w196, y=w195) -> (x != y?=w197:bool)
            n82 = Or(x=w197, y=w189) -> (x .or. y?=w187:bool)
          }
          frame "Data Information:Nanotime Gate Separation" {
            # "\"Data Information:Gate Separation\""
            n83 = call "AlliGator Settings Storage.vi"("AlliGator Settings List"=w207, "Error In"=w206) -> ("Error Out"=w204:errorcluster, "Variant Data out"=w205:variant)  [unwired: 8 in]
            n84 = Unbundle By Name(w208) -> ("Data Information.Gate Separation"=w203:dbl[unit])
            n85 = Variant To Data(error in=w204, type=w203, Variant=w205) -> (data=w202:dbl[unit], error out=w199:errorcluster)
            n86 = Not Equal?(x=w202, y=w203) -> (x != y?=w201:bool)
            n87 = Or(x=w201, y=w200) -> (x .or. y?=w198:bool)
          }
          frame "Data Information:Gate Width" {
            # "\"Data Information:Gate Width\""
            n88 = call "AlliGator Settings Storage.vi"("AlliGator Settings List"=w218, "Error In"=w217) -> ("Error Out"=w215:errorcluster, "Variant Data out"=w216:variant)  [unwired: 8 in]
            n89 = Unbundle By Name(w219) -> ("Data Information.Gate Width"=w214:dbl[unit])
            n90 = Variant To Data(error in=w215, type=w214, Variant=w216) -> (data=w213:dbl[unit], error out=w210:errorcluster)
            n91 = Not Equal?(x=w213, y=w214) -> (x != y?=w212:bool)
            n92 = Or(x=w212, y=w211) -> (x .or. y?=w209:bool)
          }
          frame "Data Information:Laser Period" {
            # "\"Data Information:Laser Period\""
            n93 = call "AlliGator Settings Storage.vi"("AlliGator Settings List"=w229, "Error In"=w228) -> ("Error Out"=w226:errorcluster, "Variant Data out"=w227:variant)  [unwired: 8 in]
            n94 = Unbundle By Name(w230) -> ("Data Information.Laser Period"=w225:dbl[unit])
            n95 = Variant To Data(error in=w226, type=w225, Variant=w227) -> (data=w224:dbl[unit], error out=w221:errorcluster)
            n96 = Not Equal?(x=w224, y=w225) -> (x != y?=w223:bool)
            n97 = Or(x=w223, y=w222) -> (x .or. y?=w220:bool)
          }
          frame "Data Information:SYNC Period" {
            # "\"Data Information:SYNC Period\""
            n98 = call "AlliGator Settings Storage.vi"("AlliGator Settings List"=w240, "Error In"=w239) -> ("Error Out"=w237:errorcluster, "Variant Data out"=w238:variant)  [unwired: 8 in]
            n99 = Unbundle By Name(w241) -> ("Data Information.SYNC Period"=w236:dbl[unit])
            n100 = Variant To Data(error in=w237, type=w236, Variant=w238) -> (data=w235:dbl[unit], error out=w232:errorcluster)
            n101 = Not Equal?(x=w235, y=w236) -> (x != y?=w234:bool)
            n102 = Or(x=w234, y=w233) -> (x .or. y?=w231:bool)
          }
          frame "Data Information:Channel Name" {
            # "\"Data Information:Channel Name\""
            n103 = call "AlliGator Settings Storage.vi"("AlliGator Settings List"=w251, "Error In"=w250) -> ("Error Out"=w248:errorcluster, "Variant Data out"=w249:variant)  [unwired: 8 in]
            n104 = Unbundle By Name(w252) -> ("Data Information.Channel Name"=w247:u16)
            n105 = Variant To Data(error in=w248, type=w247, Variant=w249) -> (data=w246:u16, error out=w243:errorcluster)
            n106 = Not Equal?(x=w246, y=w247) -> (x != y?=w245:bool)
            n107 = Or(x=w245, y=w244) -> (x .or. y?=w242:bool)
          }
          frame "Data Information:Channel Arithmetic" {
            # "\"Data Information:Channel Arithmetic\""
            n108 = call "AlliGator Settings Storage.vi"("AlliGator Settings List"=w262, "Error In"=w261) -> ("Error Out"=w259:errorcluster, "Variant Data out"=w260:variant)  [unwired: 8 in]
            n109 = Unbundle By Name(w263) -> ("Data Information.Channel Arithmetic"=w258:T14)
            n110 = Variant To Data(error in=w259, type=w258, Variant=w260) -> (data=w257:T14, error out=w254:errorcluster)
            n111 = Not Equal?(x=w257, y=w258) -> (x != y?=w256:bool)
            n112 = Or(x=w256, y=w255) -> (x .or. y?=w253:bool)
          }
          frame "Data Information:Pile-up Correction" {
            # "\"Data Information:Pile-up Correction\""
            n113 = call "AlliGator Settings Storage.vi"("AlliGator Settings List"=w273, "Error In"=w272) -> ("Error Out"=w270:errorcluster, "Variant Data out"=w271:variant)  [unwired: 8 in]
            n114 = Unbundle By Name(w274) -> ("Data Information.Pile-up Correction"=w269:bool)
            n115 = Variant To Data(error in=w270, type=w269, Variant=w271) -> (data=w268:bool, error out=w265:errorcluster)
            n116 = Not Equal?(x=w268, y=w269) -> (x != y?=w267:bool)
            n117 = Or(x=w267, y=w266) -> (x .or. y?=w264:bool)
          }
          frame "Data Information:Pixel Well Capacity" {
            # "\"Data Information:Pixel Well Capacity\""
            n118 = call "AlliGator Settings Storage.vi"("AlliGator Settings List"=w284, "Error In"=w283) -> ("Error Out"=w281:errorcluster, "Variant Data out"=w282:variant)  [unwired: 8 in]
            n119 = Unbundle By Name(w285) -> ("Data Information.Pixel Well Capacity"=w280:u32)
            n120 = Variant To Data(error in=w281, type=w280, Variant=w282) -> (data=w279:u32, error out=w276:errorcluster)
            n121 = Not Equal?(x=w279, y=w280) -> (x != y?=w278:bool)
            n122 = Or(x=w278, y=w277) -> (x .or. y?=w275:bool)
          }
          frame "Data Information:Dataset Scaling Factor" {
            # "\"Data Information:Dataset Scaling Factor\""
            n123 = call "AlliGator Settings Storage.vi"("AlliGator Settings List"=w295, "Error In"=w294) -> ("Error Out"=w292:errorcluster, "Variant Data out"=w293:variant)  [unwired: 8 in]
            n124 = Unbundle By Name(w296) -> ("Data Information.Dataset Scaling Factor"=w291:dbl)
            n125 = Variant To Data(error in=w292, type=w291, Variant=w293) -> (data=w290:dbl, error out=w287:errorcluster)
            n126 = Not Equal?(x=w290, y=w291) -> (x != y?=w289:bool)
            n127 = Or(x=w289, y=w288) -> (x .or. y?=w286:bool)
          }
          frame "Data Information:Background Scaling Factor" {
            # "\"Data Information:Background Scaling Factor\""
            n128 = call "AlliGator Settings Storage.vi"("AlliGator Settings List"=w298, "Error In"=w297) -> ("Error Out"=w306:errorcluster, "Variant Data out"=w307:variant)  [unwired: 8 in]
            n129 = Unbundle By Name(w302) -> ("Decay Preprocessing Options & Parameters.Background Subtraction Parameters.Background Scaling Factor"=w305:dbl)
            n130 = Variant To Data(error in=w306, type=w305, Variant=w307) -> (data=w304:dbl, error out=w301:errorcluster)
            n131 = Not Equal?(x=w304, y=w305) -> (x != y?=w303:bool)
            n132 = Or(x=w303, y=w300) -> (x .or. y?=w299:bool)
          }
          frame "Fluorescence Decay_Decay Pre-Processing:Background Subtraction" {
            # "\"Fluorescence Decay_Decay Pre-Processing:Background Subtraction\""
            n133 = Unbundle By Name(w313) -> ("Decay Preprocessing Options & Parameters.Background Subtraction Parameters.Background Subtraction?"=w316:bool)
            n134 = call "AlliGator Settings Storage.vi"("AlliGator Settings List"=w309, "Error In"=w308) -> ("Error Out"=w317:errorcluster, "Variant Data out"=w318:variant)  [unwired: 8 in]
            n135 = Variant To Data(error in=w317, type=w316, Variant=w318) -> (data=w315:bool, error out=w312:errorcluster)
            n136 = Not Equal?(x=w315, y=w316) -> (x != y?=w314:bool)
            n137 = Or(x=w314, y=w311) -> (x .or. y?=w310:bool)
          }
          frame "Fluorescence Decay_Decay Pre-Processing:Baseline Subtraction Method" {
            # "\"Fluorescence Decay_Decay Pre-Processing:Baseline Subtraction Method\""
            n138 = Unbundle By Name(w324) -> ("Decay Preprocessing Options & Parameters.Background Subtraction Parameters.Baseline Subtraction Method"=w327:T8)
            n139 = call "AlliGator Settings Storage.vi"("AlliGator Settings List"=w320, "Error In"=w319) -> ("Error Out"=w328:errorcluster, "Variant Data out"=w329:variant)  [unwired: 8 in]
            n140 = Variant To Data(error in=w328, type=w327, Variant=w329) -> (data=w326:T8, error out=w323:errorcluster)
            n141 = Not Equal?(x=w326, y=w327) -> (x != y?=w325:bool)
            n142 = Or(x=w325, y=w322) -> (x .or. y?=w321:bool)
          }
          frame "Fluorescence Decay_Decay Pre-Processing:Background Definition Range" {
            # "\"Fluorescence Decay_Decay Pre-Processing:Background Definition Range\""
            n143 = call "AlliGator Settings Storage.vi"("AlliGator Settings List"=w331, "Error In"=w330) -> ("Error Out"=w339:errorcluster, "Variant Data out"=w340:variant)  [unwired: 8 in]
            n144 = Unbundle By Name(w335) -> ("Decay Preprocessing Options & Parameters.Background Subtraction Parameters.Background Definition Range"=w338:T23)
            n145 = Variant To Data(error in=w339, type=w338, Variant=w340) -> (data=w337:T23, error out=w334:errorcluster)
            n146 = Not Equal?(x=w337, y=w338) -> (x != y?=w336:bool)
            n147 = Or(x=w336, y=w333) -> (x .or. y?=w332:bool)
          }
          frame "Fluorescence Decay_Decay Pre-Processing:Constant Background" {
            # "\"Fluorescence Decay_Decay Pre-Processing:Constant Background\""
            n148 = call "AlliGator Settings Storage.vi"("AlliGator Settings List"=w342, "Error In"=w341) -> ("Error Out"=w350:errorcluster, "Variant Data out"=w351:variant)  [unwired: 8 in]
            n149 = Unbundle By Name(w346) -> ("Decay Preprocessing Options & Parameters.Background Subtraction Parameters.Background Constant"=w349:dbl)
            n150 = Variant To Data(error in=w350, type=w349, Variant=w351) -> (data=w348:dbl, error out=w345:errorcluster)
            n151 = Not Equal?(x=w348, y=w349) -> (x != y?=w347:bool)
            n152 = Or(x=w347, y=w344) -> (x .or. y?=w343:bool)
          }
          frame "Fluorescence Decay_Decay Pre-Processing:Decay Pre-Processing Operations Order" {
            # "\"Fluorescence Decay_Decay Pre-Processing:Decay Pre-Processing Operations Order\""
            n153 = call "AlliGator Settings Storage.vi"("AlliGator Settings List"=w353, "Error In"=w352) -> ("Error Out"=w361:errorcluster, "Variant Data out"=w362:variant)  [unwired: 8 in]
            n154 = Unbundle By Name(w357) -> ("Decay Preprocessing Options & Parameters.Preprocessing Steps Order"=w360:string[])
            n155 = Variant To Data(error in=w361, type=w360, Variant=w362) -> (data=w359:string[], error out=w356:errorcluster)
            n156 = Not Equal?(x=w359, y=w360) -> (x != y?=w358:bool)
            n157 = Or(x=w358, y=w355) -> (x .or. y?=w354:bool)
          }
          frame "Miscellaneous:Verbose Error Mode" {
            # "Miscellaneous:Verbose Error Mode: This is used as a placeholder for Decay Preprocessing Parameters"
            n158 = Unbundle By Name(w369) -> ("Decay Preprocessing Options & Parameters.Decay Preprocessing Parameters"=w371:T9)
            n159 = call "AlliGator Get-Set Decay Preprocessing Parameters.vi"("Get (F)/Set"=FALSE, "Error In"=w365) -> ("Error Out"=w364:errorcluster, "Decay Preprocessing Parameters out"=w366:T9)  [unwired: 8 in]
            n160 = Not Equal?(x=w366, y=w371) -> (x != y?=w370:bool)
            n161 = Or(x=w370, y=w368) -> (x .or. y?=w367:bool)
          }
          frame "Miscellaneous:Verbose Settings Mode" {
            # "Miscellaneous:Verbose Settings Mode: This is used as a placeholder for FLI Dataset Modified"
            n162 = call "Alligator Variables Storage.vi"("AlliGator Variable"=AlliGator_Variables_List."Phasor Plot:FLI Dataset Modified since last Calculation" ("Alligator Variable"), "Error In"=w376) -> ("Error Out"=w377:errorcluster, "Data out"=w374:variant)  [unwired: 7 in, 1 out]
            n163 = call-poly "Variant to Data.vi"("Variant"=w374) -> ("Value"=w373:bool)  [unwired: 8 in]
            n164 = Unbundle By Name(w380) -> ("FLI Dataset Modified"=w372:bool)
            n165 = Not Equal?(x=w373, y=w372) -> (x != y?=w381:bool)
            n166 = Or(x=w381, y=w379) -> (x .or. y?=w378:bool)
          }
        }
      }
      n167 = Merge Errors(w26) -> (w25:errorcluster)
      n168 = call "AlliGator Set Phasor Plot Update LED.vi"("error in (no error)"=w25, "Off/On"=w24) -> ("error out"=w30:errorcluster)  [unwired: 9 in]
    }
  }
  "Error Out" <- w19
